vi "Replace Line.vi"(8 "error in":errorcluster, 9 "New Line":T1, 10 "Line Name":string, 11 "FPGA Module configuration in":refnum<class "FPGA Module configuration.lvclass">) -> (0 "error out":errorcluster, 2 "Old Line":T1, 3 "FPGA Module configuration out":refnum<class "FPGA Module configuration.lvclass">)   [LabVIEW 2013, in "FPGA Module configuration.lvclass"]
doc: "Replaces a line identified by name with a new line."
uses:
  FPGA Module configuration.lvclass
  Line.ctl
  <vilib>/NI/Tag Bus Module Framework/channel/TBM channel.lvclass
  FPGA Module configuration.lvclass/FPGA Module configuration.ctl
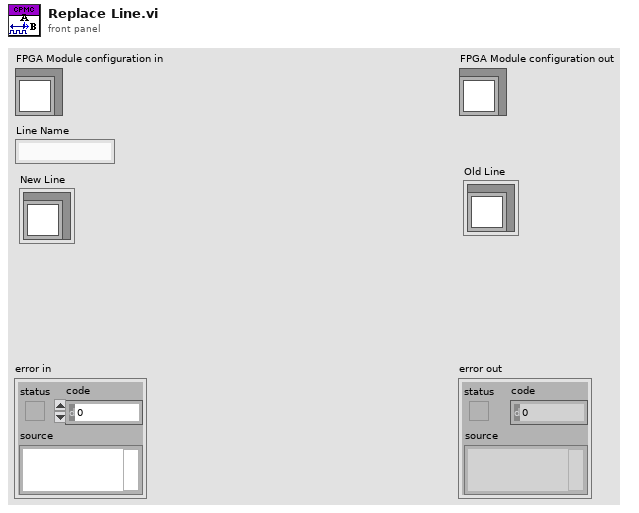
[diagram p1: front panel]
types:
  T1 = typedef "FPGA Module configuration.lvclass/Line.ctl" = cluster{"channel":refnum<class "TBM channel.lvclass">}
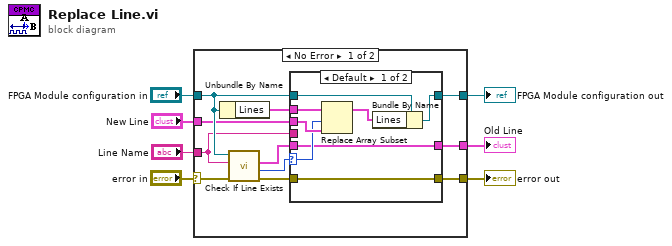
[diagram p0: block diagram]
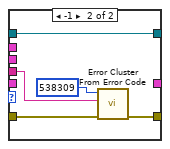
[diagram p2: hidden frame]
diagram:
  n1 = case shown="No Error" "error in" {
    selector: "error in" -> [w10 w33]
    tunnel: [w17 w33] -> w6
    tunnel: [w18 w32] -> w4
    tunnel: "FPGA Module configuration in" -> [w16 w32]
    tunnel: "Line Name" -> [w15 _]
    tunnel: "New Line" -> [w13 _]
    tunnel: [w11 _] -> w1
    frame No Error {
      n2 = Unbundle By Name(w16) -> ("Lines"=w12:T1[])
      n3 = call-dynamic "Check If Line Exists.vi"("error in"=w10, "Name to Locate"=w15, "FPGA Module configuration in"=w16) -> ("error out"=w9:errorcluster, "Index"=w14:i32, "Line out"=w8:T1)  [unwired: 4 in, 2 out]
      n4 = case shown="Default" w14 {
        selector: w14 -> [w20 _]
        tunnel: w16 -> [w26 w31]
        tunnel: [w25 w31] -> w18
        tunnel: w12 -> [w21 _]
        tunnel: w13 -> [w23 _]
        tunnel: w15 -> [_ w29]
        tunnel: w9 -> [w22 w28]
        tunnel: [w22 w27] -> w17
        tunnel: [w19 _] -> w11
        tunnel: w8 -> [w19 _]
        frame Default {
          n5 = Replace Array Subset(array=w21, new element=w23, index=w20) -> (w24:T1[])
          n6 = Bundle By Name(cluster=w26, "Lines"=w24) -> (w25:refnum<class "FPGA Module configuration.lvclass">)
        }
        frame -1 {
          n7 = call <vilib>:"Error Cluster From Error Code.vi"("error in (no error)"=w28, "error message (\"\")"=w29, "error code (0)"=538309) -> ("error out"=w27:errorcluster)  [unwired: 6 in]
        }
      }
    }
    frame Error {
    }
  }
  "error out" <- w6
  "FPGA Module configuration out" <- w4
  "Old Line" <- w1
